vi "DrainAndBlow.vi"(11 "LWSR":refnum<class "Web Request.lvclass">) -> ()   [LabVIEW 2019]
uses:
  <vilib>/wsapi/Web Request.lvclass
panel:
  out "postdata":string
  out "number":i32
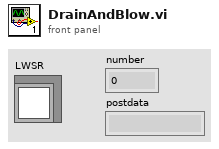
[diagram p1: front panel]
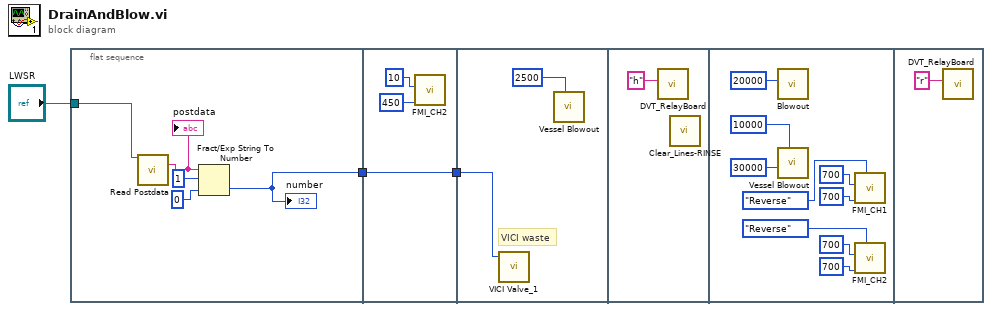
[diagram p0: block diagram]
diagram:
  n1 = flat-sequence {
    tunnel: [w6] -> w2
    tunnel: "LWSR" -> [w4]
    tunnel: w2 -> [w9]
    tunnel: [w9] -> w1
    tunnel: w1 -> [w12]
    frame #0 {
      n2 = call <vilib>:"Read Postdata.vi"("LabVIEW Web Service Request"=w4) -> ("postdata"=w7:string)  [unwired: 12 in, 2 out]
      "postdata" <- w7
      n3 = Fract/Exp String To Number(string=w7, offset=1, default (0 dbl)=0 ("default (0 DBL)")) -> (number=w6:i32)  [unwired: 1 in, 1 out]
      "number" <- w6
    }
    frame #1 {
      n4 = call "FMI_CH2.vi"("RPM"=450, "Strokes"=10) -> ()  [unwired: 6 in]
    }
    frame #2 {
      # "VICI waste"
      n5 = call "VICI Valve_1.vi"("RequestedValve#"=w12) -> ()  [unwired: 2 in, 3 out]
      n6 = call "Vessel Blowout.vi"("Blowtime(ms)"=u32 2500 ("Mixtime(ms)")) -> ()  [unwired: 11 in]
    }
    frame #3 {
      n7 = call "DVT_RelayBoard.vi"("write buffer"="h") -> ()  [unwired: 3 in, 3 out]
      n8 = call "Clear_Lines-RINSE.vi"() -> ()  [unwired: 12 in]
    }
    frame #4 {
      n9 = call "Blowout.vi"("Blowout (ms)"=u32 20000) -> ()  [unwired: 11 in]
      n10 = call "Vessel Blowout.vi"("Blowtime(ms)"=u32 10000 ("Mixtime(ms)"), "Delay(ms)"=u32 30000) -> ()  [unwired: 10 in]
      n11 = call "FMI_CH1.vi"("Direction"=enum16{"Forward", "Reverse"}."Reverse", "RPM"=700, "Strokes"=700) -> ()  [unwired: 5 in]
      n12 = call "FMI_CH2.vi"("Direction"=enum16{"Forward", "Reverse"}."Reverse", "RPM"=700, "Strokes"=700) -> ()  [unwired: 5 in]
    }
    frame #5 {
      n13 = call "DVT_RelayBoard.vi"("write buffer"="r") -> ()  [unwired: 3 in, 3 out]
    }
  }
